vi "testUnflattenTemperatureAbsFromXML.vi"() -> ()   [LabVIEW 2012, in "UnitsAndXML.lvlib"]
uses:
  <userlib>/Common/UnitsAndXML/UnitsAndXML.lvlib
  <userlib>/Common/UnitsAndXML/FlattenItemWithUnitToXML/FlattenTemperatureAbsToXML/TemperatureAbsUnit.ctl
  <userlib>/Common/UnitsAndXML/UnflattenItemWithUnitFromXML/UnflattenTemperatureAbsFromXML/typeMethods/unflattenTemperatureAbsFromXML_Array.vi
  <userlib>/Common/UnitsAndXML/UnflattenItemWithUnitFromXML/UnflattenTemperatureAbsFromXML/typeMethods/unflattenTemperatureAbsFromXML_Scalar.vi
panel:
  out "error out":errorcluster
  out "temperatureAbs":dbl[unit][](array[numeric])
  out "time":dbl[unit]=273.15
  in  "temperatureAbsUnitInXML":T1
  in  "xmlStringArray":string="<temperatureAbs>15</temperatureAbs>\r\n<temperatureAbs>30</temperatureAbs>\r\n<temperatureAbs>45</temperatureAbs>\r\n<temperatureAbs>60</temperatureAbs>"
  in  "xmlStringScalar":string="<temperatureAbs>15</temperatureAbs>"
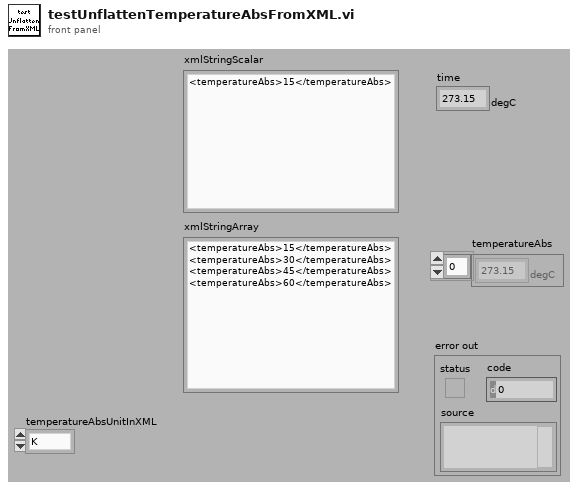
[diagram p1: front panel]
types:
  T1 = typedef "UnitsAndXML.lvlib/TemperatureAbsUnit.ctl" = enum16{"K", "degC", "degF"}
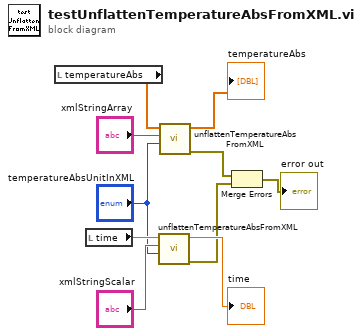
[diagram p0: block diagram]
diagram:
  n1 = local read "temperatureAbs"() -> (w3:dbl[unit][])
  n2 = local read "time"() -> (w9:dbl[unit])
  n3 = call-poly <userlib>:"unflattenTemperatureAbsFromXML.vi"("temperatureAbsUnitInXML"="temperatureAbsUnitInXML", "xmlString"="xmlStringScalar", "temperatureAbsForType"=w9) -> ("error out"=w5:errorcluster, "temperatureAbs"=→"time":dbl[unit])  [unwired: 7 in]
  n4 = call-poly <userlib>:"unflattenTemperatureAbsFromXML.vi"("temperatureAbsUnitInXML"="temperatureAbsUnitInXML", "xmlString"="xmlStringArray", "temperatureAbsForType"=w3) -> ("error out"=w6:errorcluster, "temperatureAbs"=→"temperatureAbs":dbl[unit][])  [unwired: 7 in]
  n5 = Merge Errors(w6, w5) -> (→"error out":errorcluster)
